vi "FrameCycling.vi"(5 "Skip":bool, 7 "Pause":bool, 8 "Skip to Frame":i32, 9 "Total Reel Frames":i32, 10 "Current Frame":i32, 11 "Animation Reel In":picture[](array[picture])) -> (0 "Frame Output":picture, 2 "Next Fame":i32, 3 "Animation Reel Out":picture[](array[picture]))   [LabVIEW 2014]
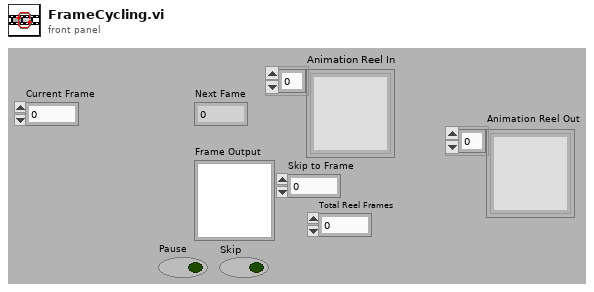
[diagram p1: front panel]
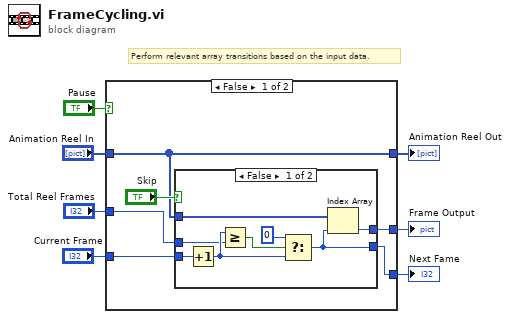
[diagram p0: block diagram]
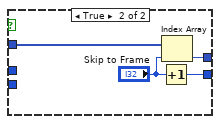
[diagram p2: hidden frame]
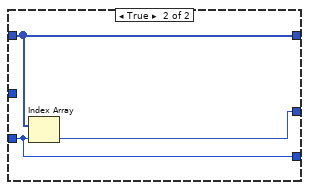
[diagram p3: hidden frame]
diagram:
  # "Perform relevant array transitions based on the input data."
  n1 = case shown="False" "Pause" {
    tunnel: [w13 w26] -> w7
    tunnel: "Current Frame" -> [w12 w26]
    tunnel: "Animation Reel In" -> [w8 w28]
    tunnel: [w8 w28] -> w3
    tunnel: [w11 w27] -> w2
    tunnel: "Total Reel Frames" -> [w10 _]
    frame False {
      n2 = case shown="False" "Skip" {
        tunnel: [w17 w23] -> w13
        tunnel: w12 -> [w16 _]
        tunnel: w8 -> [w19 w25]
        tunnel: [w18 w24] -> w11
        tunnel: w10 -> [w14 _]
        frame False {
          n3 = Increment(x=w16) -> (x+1=w15:i32)
          n4 = Greater Or Equal?(x=w15, y=w14) -> (x >= y?=w20:bool)
          n5 = Select(t=0, s=w20, f=w15) -> (s? t:f=w17:i32)
          n6 = Index Array(array=w19, index=w17) -> (element=w18:picture)
        }
        frame True {
          n7 = Increment(x="Skip to Frame") -> (x+1=w23:i32)
          n8 = Index Array(array=w25, index="Skip to Frame") -> (element=w24:picture)
        }
      }
    }
    frame True {
      n9 = Index Array(array=w28, index=w26) -> (element=w27:picture)
    }
  }
  "Next Fame" <- w7
  "Animation Reel Out" <- w3
  "Frame Output" <- w2
